vi "Close.vi"(8 "error in (no error)":errorcluster, 11 "NI DIO in":refnum<class "NI DIO.lvclass">) -> (0 "error out":errorcluster, 3 "NI DIO out":refnum<class "NI DIO.lvclass">)   [LabVIEW 2025, in "Digital IO.lvlib" / "NI DIO.lvclass"]
uses:
  NI DIO.lvclass
  NI DIO.lvclass/NI DIO.ctl
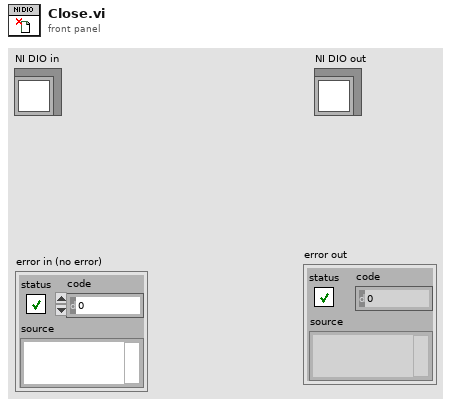
[diagram p1: front panel]
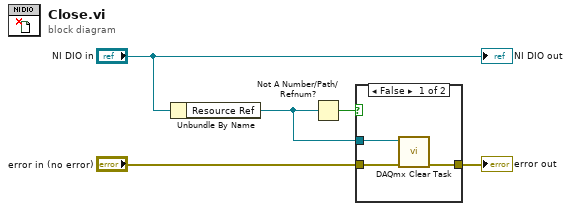
[diagram p0: block diagram]
diagram:
  n1 = Unbundle By Name("NI DIO in") -> ("Resource Ref"=w1:refnum<k21>)
  n2 = Not A Number/Path/Refnum?(number/path/refnum=w1) -> (NaN/Path/Refnum?=w2:bool)
  n3 = case shown="False" w2 {
    tunnel: "error in (no error)" -> [w8 w9]
    tunnel: [w7 w9] -> w3
    tunnel: w1 -> [w6 _]
    frame False {
      n4 = call <vilib>:"DAQmx Clear Task.vi"("task in"=w6, "error in"=w8) -> ("error out"=w7:errorcluster)  [unwired: 13 in]
    }
    frame True {
    }
  }
  "error out" <- w3
  "NI DIO out" <- "NI DIO in"
